vi "get fpga resource ref from ctrl name.vi"(8 "error in (no error)":errorcluster, 9 "Data type":variant, 10 "Resource name":string, 11 "Refnum in":refnum<k20>) -> (0 "error out":errorcluster, 1 "FXP type supported":bool, 2 "fpga res type":T1, 3 "Refnum out":refnum<k20>)   [LabVIEW 2015]
uses:
  configuration/fpga resource supported data types.ctl
  FXP I_20_5.ctl
  FXP I_24_5.ctl
  FXP I_24_10.ctl
  <vilib>/NI/LVFPGA Adv Session Resources/OpenByNameSubVI.vi
  <vilib>/rvi/interface/common/dynamic/niFpgaEscapeDelimiterAndNull.vi
  <vilib>/Utility/error.llb/Error Cluster From Error Code.vi
  <vilib>/rvi/interface/common/niFpgaWaitOnOcc.vi
  <vilib>/NI/LVFPGA Adv Session Resources/OpenByName.xnode
  <vilib>/rvi/interface/nirviMethod/nirviMethod.xnode
  configuration/io configuration.lvclass
  <vilib>/NI/LVFPGA Adv Session Resources/LVFPGAAdvSessionResources.lvlib
  <vilib>/Utility/Data Type/NI_Data Type.lvlib
  io runtime.lvclass
  <vilib>/rvi/errors/niLvFpgaMergeErrorWithErrorCode.vi
  <vilib>/FPGAPlugInAG/Dynamic/niLvFpga_ConfigureFifo_Dynamic.vi
  <vilib>/FPGAPlugInAG/Dynamic/niLvFpga_StartFifo_Dynamic.vi
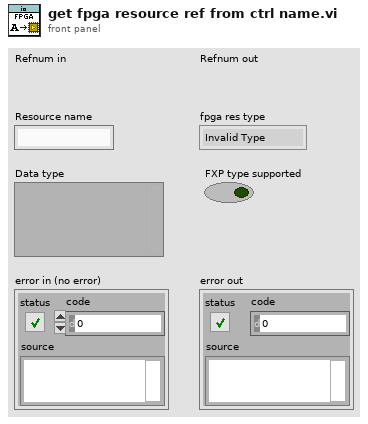
[diagram p1: front panel]
types:
  T1 = typedef "io configuration.lvclass/fpga resource supported data types.ctl" = enum16{"Invalid Type", "Single", "I64", "I32", "I16", "I8", "U64", "U32", "U16", "U8", "Boolean", "FXP I,20,5", "FXP I,24,5", "FXP I,24,10", "Fifo 1023,I16"}
  T2 = typedef "NI_Data Type.lvlib/Data Type.ctl" = enum8{"Invalid Type", "Void", "I8", "I16", "I32", "I64", "U8", "U16", "U32", "U64", "Single Float", "Double Float", "Extended Float", "Single Complex", "Double Complex", "Extended Complex", "Enum U8", "Enum U16", "Enum U32", "Enum U64", "Single Float With Unit", "Double Float With Unit", "Extended Float With Unit", "Single Complex with Unit", "Double Complex with Unit", "Extended Complex with Unit", "Boolean", "String", "Path", "Picture", "Tag", "Array", "Cluster", "Variant", "LV Variant", "Waveform", "Timestamp", "Digital Waveform", "Digital Data", "ExpressData", "Refnum", "External Data", "VI", "Poly VI", "LabVIEW Class Instance", "Fixed Point"}
  T3 = cluster{"Name":string, "Depth":u32, "Write? (Deprecated:Use Implementation)":bool, "Physical Channel":u32, "Base Address":u32, "Data Width":u32, "Data Type":enum32{"Boolean", "I8", "I16", "I32", "I64", "U8", "U16", "U32", "U64", "FXP", "CustomControl", "SGL"}, "FXP Properties":variant, "Write Window Address":u32, "Implementation":enum16{"niFpgaTargetToHost", "niFpgaHostToTarget", "niFpgaPeerToPeerWriter", "niFpgaPeerToPeerReader", "niCoreTargetToHost", "niCoreHostToTarget"}, "Control Set":u32}[]
  T4 = cluster{"Name":string, "type":variant, "indicator?":bool}[]
  T5 = typedef "LVFixedPointRepBitsTypeDef.ctl" = cluster{"Signed":bool, "Word Length":u32, "Integer Word Length":i32}
  T6 = typedef "io runtime.lvclass/FXP I_20_5.ctl" = refnum<k20>
  T7 = typedef "io runtime.lvclass/FXP I_24_5.ctl" = refnum<k20>
  T8 = typedef "io runtime.lvclass/FXP I_24_10.ctl" = refnum<k20>
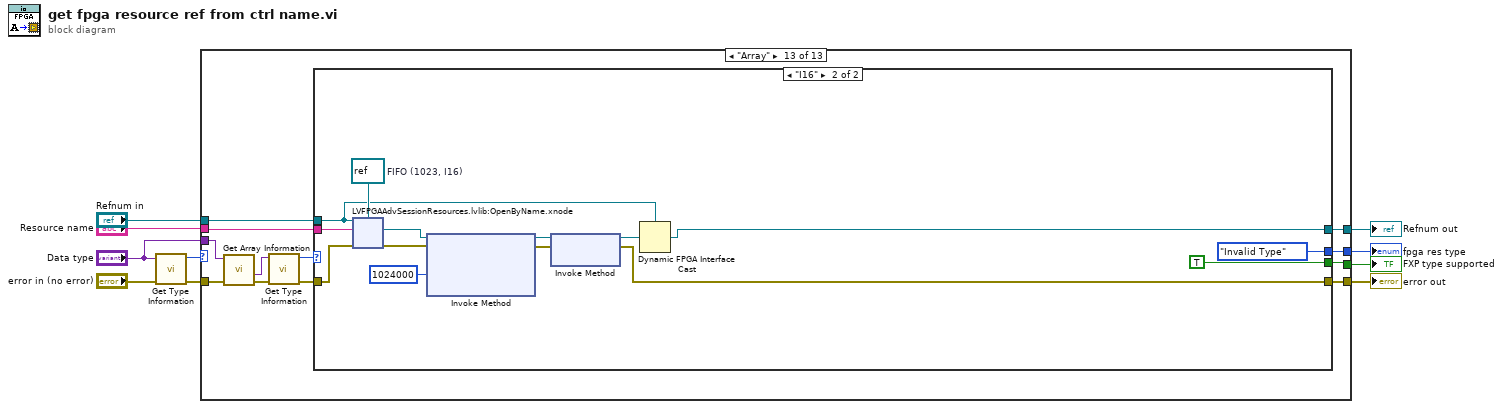
[diagram p0: block diagram]
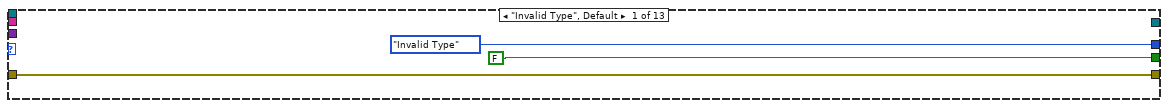
[diagram p2: hidden frame]
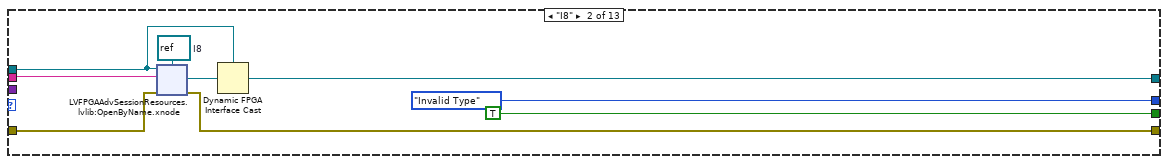
[diagram p3: hidden frame]
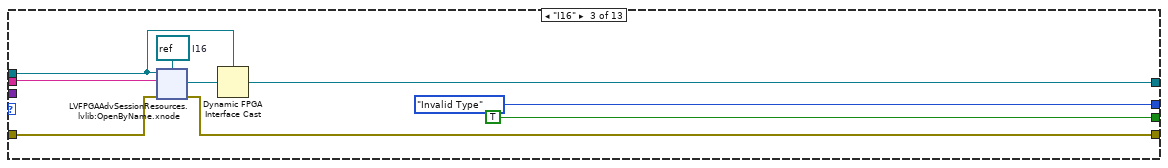
[diagram p4: hidden frame]
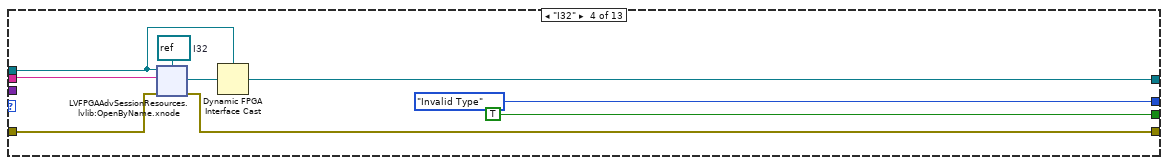
[diagram p5: hidden frame]
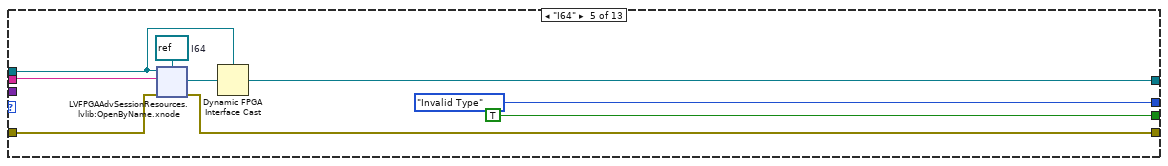
[diagram p6: hidden frame]
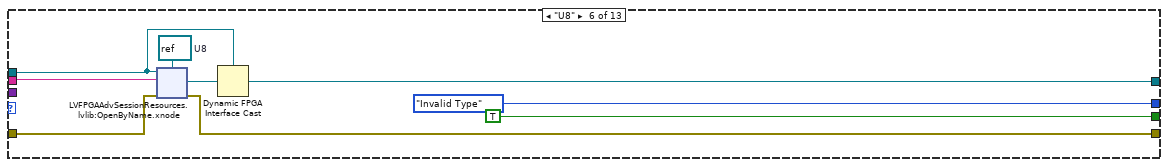
[diagram p7: hidden frame]
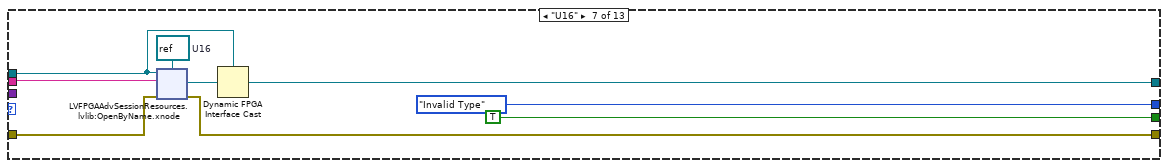
[diagram p8: hidden frame]
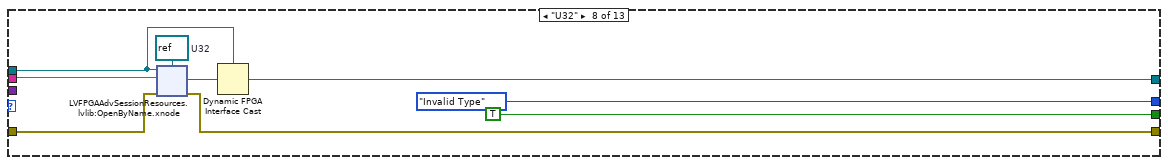
[diagram p9: hidden frame]
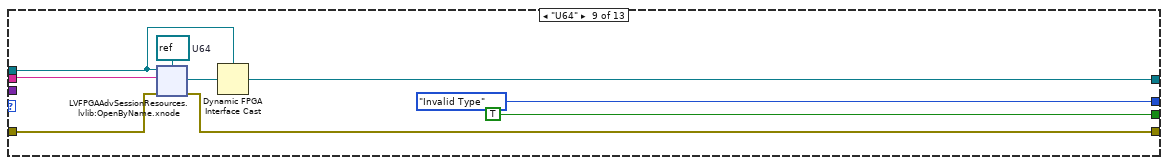
[diagram p10: hidden frame]
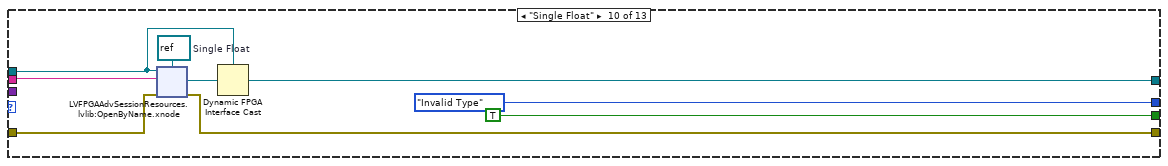
[diagram p11: hidden frame]
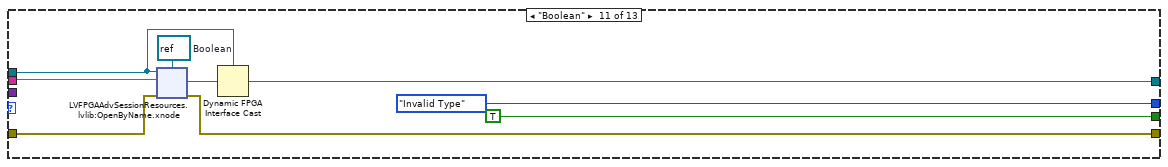
[diagram p12: hidden frame]
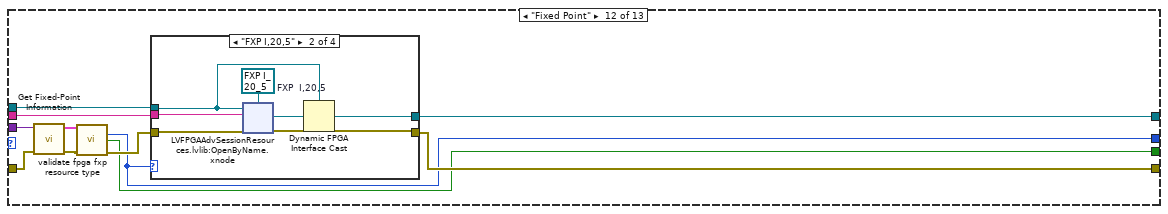
[diagram p13: hidden frame]
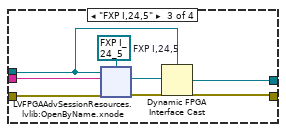
[diagram p15: hidden frame]
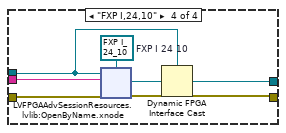
[diagram p16: hidden frame]
diagram:
  n1 = call <vilib>:"Get Type Information.vi"("error in (no error)"="error in (no error)", "Variant"="Data type") -> ("error out"=w2:errorcluster, "Type"=w1:T2)  [unwired: 5 in, 3 out]
  n2 = case shown="\"Array\"" w1 {
    tunnel: w2 -> [w12 w19 w42 w64 w86 w108 w130 w152 w174 w196 w218 w243 w314]
    tunnel: [FALSE TRUE TRUE TRUE TRUE TRUE TRUE TRUE TRUE TRUE TRUE w234 w312] -> w8
    tunnel: [w12 w18 w41 w63 w85 w107 w129 w151 w173 w195 w217 w237 w308] -> w9
    tunnel: "Data type" -> [_ _ _ _ _ _ _ _ _ _ _ w244 w313]
    tunnel: "Resource name" -> [_ w17 w40 w62 w84 w106 w128 w150 w172 w194 w216 w239 w307]
    tunnel: "Refnum in" -> [_ w16 w39 w61 w83 w105 w127 w149 w171 w193 w215 w240 w311]
    tunnel: [_ w15 w38 w60 w82 w104 w126 w148 w170 w192 w214 w236 w309] -> w7
    tunnel: [fpga_resource_supported_data_types."Invalid Type" ("fpga res type") fpga_resource_supported_data_types."Invalid Type" ("fpga res type") fpga_resource_supported_data_types."Invalid Type" ("fpga res type") fpga_resource_supported_data_types."Invalid Type" ("fpga res type") fpga_resource_supported_data_types."Invalid Type" ("fpga res type") fpga_resource_supported_data_types."Invalid Type" ("fpga res type") fpga_resource_supported_data_types."Invalid Type" ("fpga res type") fpga_resource_supported_data_types."Invalid Type" ("fpga res type") fpga_resource_supported_data_types."Invalid Type" ("fpga res type") fpga_resource_supported_data_types."Invalid Type" ("fpga res type") fpga_resource_supported_data_types."Invalid Type" ("fpga res type") w235 w306] -> w6
    frame "Invalid Type", Default {
    }
    frame "I8" {
      w20 = refnum<k20> refnum  # I8
      n3 = xnode "LVFPGAAdvSessionResources.lvlib:OpenByName.xnode"("FPGA VI Reference in"=w16, "Resource name in"=w17, "Single resource reference type in"=w20, "Error in"=w19) -> ("Single resource reference out"=w21:refnum<k20>, "Error out"=w18:errorcluster)  [unwired: 1 out]
      n4 = Dynamic FPGA Interface Cast(Session In=w16, Type=w21) -> (Session Out=w15:refnum<k20>)
    }
    frame "I16" {
      w36 = refnum<k20> refnum  # I16
      n5 = xnode "LVFPGAAdvSessionResources.lvlib:OpenByName.xnode"("FPGA VI Reference in"=w39, "Resource name in"=w40, "Single resource reference type in"=w36, "Error in"=w42) -> ("Single resource reference out"=w43:refnum<k20>, "Error out"=w41:errorcluster)  [unwired: 1 out]
      n6 = Dynamic FPGA Interface Cast(Session In=w39, Type=w43) -> (Session Out=w38:refnum<k20>)
    }
    frame "I32" {
      w58 = refnum<k20> refnum  # I32
      n7 = xnode "LVFPGAAdvSessionResources.lvlib:OpenByName.xnode"("FPGA VI Reference in"=w61, "Resource name in"=w62, "Single resource reference type in"=w58, "Error in"=w64) -> ("Single resource reference out"=w65:refnum<k20>, "Error out"=w63:errorcluster)  [unwired: 1 out]
      n8 = Dynamic FPGA Interface Cast(Session In=w61, Type=w65) -> (Session Out=w60:refnum<k20>)
    }
    frame "I64" {
      w80 = refnum<k20> refnum  # I64
      n9 = xnode "LVFPGAAdvSessionResources.lvlib:OpenByName.xnode"("FPGA VI Reference in"=w83, "Resource name in"=w84, "Single resource reference type in"=w80, "Error in"=w86) -> ("Single resource reference out"=w87:refnum<k20>, "Error out"=w85:errorcluster)  [unwired: 1 out]
      n10 = Dynamic FPGA Interface Cast(Session In=w83, Type=w87) -> (Session Out=w82:refnum<k20>)
    }
    frame "U8" {
      w102 = refnum<k20> refnum  # U8
      n11 = xnode "LVFPGAAdvSessionResources.lvlib:OpenByName.xnode"("FPGA VI Reference in"=w105, "Resource name in"=w106, "Single resource reference type in"=w102, "Error in"=w108) -> ("Single resource reference out"=w109:refnum<k20>, "Error out"=w107:errorcluster)  [unwired: 1 out]
      n12 = Dynamic FPGA Interface Cast(Session In=w105, Type=w109) -> (Session Out=w104:refnum<k20>)
    }
    frame "U16" {
      w124 = refnum<k20> refnum  # U16
      n13 = xnode "LVFPGAAdvSessionResources.lvlib:OpenByName.xnode"("FPGA VI Reference in"=w127, "Resource name in"=w128, "Single resource reference type in"=w124, "Error in"=w130) -> ("Single resource reference out"=w131:refnum<k20>, "Error out"=w129:errorcluster)  [unwired: 1 out]
      n14 = Dynamic FPGA Interface Cast(Session In=w127, Type=w131) -> (Session Out=w126:refnum<k20>)
    }
    frame "U32" {
      w146 = refnum<k20> refnum  # U32
      n15 = xnode "LVFPGAAdvSessionResources.lvlib:OpenByName.xnode"("FPGA VI Reference in"=w149, "Resource name in"=w150, "Single resource reference type in"=w146, "Error in"=w152) -> ("Single resource reference out"=w153:refnum<k20>, "Error out"=w151:errorcluster)  [unwired: 1 out]
      n16 = Dynamic FPGA Interface Cast(Session In=w149, Type=w153) -> (Session Out=w148:refnum<k20>)
    }
    frame "U64" {
      w168 = refnum<k20> refnum  # U64
      n17 = xnode "LVFPGAAdvSessionResources.lvlib:OpenByName.xnode"("FPGA VI Reference in"=w171, "Resource name in"=w172, "Single resource reference type in"=w168, "Error in"=w174) -> ("Single resource reference out"=w175:refnum<k20>, "Error out"=w173:errorcluster)  [unwired: 1 out]
      n18 = Dynamic FPGA Interface Cast(Session In=w171, Type=w175) -> (Session Out=w170:refnum<k20>)
    }
    frame "Single Float" {
      w190 = refnum<k20> refnum  # Single Float
      n19 = xnode "LVFPGAAdvSessionResources.lvlib:OpenByName.xnode"("FPGA VI Reference in"=w193, "Resource name in"=w194, "Single resource reference type in"=w190, "Error in"=w196) -> ("Single resource reference out"=w197:refnum<k20>, "Error out"=w195:errorcluster)  [unwired: 1 out]
      n20 = Dynamic FPGA Interface Cast(Session In=w193, Type=w197) -> (Session Out=w192:refnum<k20>)
    }
    frame "Boolean" {
      w212 = refnum<k20> refnum  # Boolean
      n21 = xnode "LVFPGAAdvSessionResources.lvlib:OpenByName.xnode"("FPGA VI Reference in"=w215, "Resource name in"=w216, "Single resource reference type in"=w212, "Error in"=w218) -> ("Single resource reference out"=w219:refnum<k20>, "Error out"=w217:errorcluster)  [unwired: 1 out]
      n22 = Dynamic FPGA Interface Cast(Session In=w215, Type=w219) -> (Session Out=w214:refnum<k20>)
    }
    frame "Fixed Point" {
      n23 = call <vilib>:"Get Fixed-Point Information.vi"("error in (no error)"=w243, "Variant"=w244) -> ("error out"=w242:errorcluster, "FXP Representation"=w241:T5)  [unwired: 6 in, 2 out]
      n24 = call "validate fpga fxp resource type.vi"("FXP Representation"=w241, "error in (no error)"=w242) -> ("fpga res type"=w235:T1, "FXP type supported"=w234:bool, "error out"=w238:errorcluster)  [unwired: 11 in]
      n25 = case shown="\"FXP I,20,5\"" w235 {
        tunnel: w240 -> [_ w247 w272 w291]
        tunnel: [_ w251 w271 w290] -> w236
        tunnel: w239 -> [_ w250 w270 w289]
        tunnel: w238 -> [w245 w249 w269 w288]
        tunnel: [w245 w248 w268 w287] -> w237
        frame "Invalid Type", Default {
        }
        frame "FXP I,20,5" {
          w246 = T6 refnum  # FXP  I,20,5
          n26 = xnode "LVFPGAAdvSessionResources.lvlib:OpenByName.xnode"("FPGA VI Reference in"=w247, "Resource name in"=w250, "Single resource reference type in"=w246, "Error in"=w249) -> ("Single resource reference out"=w252:T6, "Error out"=w248:errorcluster)  [unwired: 1 out]
          n27 = Dynamic FPGA Interface Cast(Session In=w247, Type=w252) -> (Session Out=w251:refnum<k20>)
        }
        frame "FXP I,24,5" {
          w266 = T7 refnum  # FXP I,24,5
          n28 = xnode "LVFPGAAdvSessionResources.lvlib:OpenByName.xnode"("FPGA VI Reference in"=w272, "Resource name in"=w270, "Single resource reference type in"=w266, "Error in"=w269) -> ("Single resource reference out"=w267:T7, "Error out"=w268:errorcluster)  [unwired: 1 out]
          n29 = Dynamic FPGA Interface Cast(Session In=w272, Type=w267) -> (Session Out=w271:refnum<k20>)
        }
        frame "FXP I,24,10" {
          w286 = T8 refnum  # FXP I 24 10
          n30 = xnode "LVFPGAAdvSessionResources.lvlib:OpenByName.xnode"("FPGA VI Reference in"=w291, "Resource name in"=w289, "Single resource reference type in"=w286, "Error in"=w288) -> ("Single resource reference out"=w292:T8, "Error out"=w287:errorcluster)  [unwired: 1 out]
          n31 = Dynamic FPGA Interface Cast(Session In=w291, Type=w292) -> (Session Out=w290:refnum<k20>)
        }
      }
    }
    frame "Array" {
      n32 = call <vilib>:"Get Array Information.vi"("error in (no error)"=w314, "Variant"=w313) -> ("error out"=w316:errorcluster, "Array Element Data Type"=w315:variant)  [unwired: 6 in, 2 out]
      n33 = call <vilib>:"Get Type Information.vi"("error in (no error)"=w316, "Variant"=w315) -> ("error out"=w310:errorcluster, "Type"=w317:T2)  [unwired: 5 in, 3 out]
      n34 = case shown="\"I16\"" w317 {
        tunnel: [_ TRUE] -> w312
        tunnel: w311 -> [_ w324]
        tunnel: w310 -> [w318 w326]
        tunnel: [_ w323] -> w309
        tunnel: [w318 w322] -> w308
        tunnel: w307 -> [_ w320]
        tunnel: [_ fpga_resource_supported_data_types."Invalid Type" ("fpga res type")] -> w306
        frame "Invalid Type", Default {
        }
        frame "I16" {
          w327 = refnum<k20> refnum  # FIFO (1023, I16)
          n35 = xnode "LVFPGAAdvSessionResources.lvlib:OpenByName.xnode"("FPGA VI Reference in"=w324, "Resource name in"=w320, "Single resource reference type in"=w327, "Error in"=w326) -> ("Single resource reference out"=w321:refnum<k20>, "Error out"=w330:errorcluster)  [unwired: 1 out]
          n36 = xnode "Invoke Method"("FPGA VI Reference In"=w321, "error in"=w330, "Requested Depth"=u32 1024000) -> ("FPGA VI Reference Out"=w328:refnum<k20>, "error out"=w329:errorcluster)  [unwired: 1 out]
          n37 = xnode "Invoke Method"("FPGA VI Reference In"=w328, "error in"=w329) -> ("FPGA VI Reference Out"=w325:refnum<k20>, "error out"=w322:errorcluster)
          n38 = Dynamic FPGA Interface Cast(Session In=w324, Type=w325) -> (Session Out=w323:refnum<k20>)
        }
      }
    }
  }
  "error out" <- w9
  "FXP type supported" <- w8
  "Refnum out" <- w7
  "fpga res type" <- w6
